vi "Initialize Hardware.vi"(8 "error in (no error)":errorcluster, 9 "Connection Setting":T1={"Connection Ref"=variant, "Serial Configuration"={"Baud Rate"=9600}} {"Serial Configuration"."Baud Rate" items=["300"=300, "600"=600, "1200"=1200, "2400"=2400, "4800"=4800, "9600"=9600, "19200"=19200]}, 10 "DAQ Type":enum16{"Hardware", "Simulation"}(ring), 11 "BK-Precision in":refnum<class "BK-Precision.lvclass">) -> (0 "error out":errorcluster, 3 "BK-Precision out":refnum<class "BK-Precision.lvclass">)   [LabVIEW 2021, in "DC PWS.lvlib" / "BK-Precision.lvclass"]
uses:
  BK-Precision.lvclass
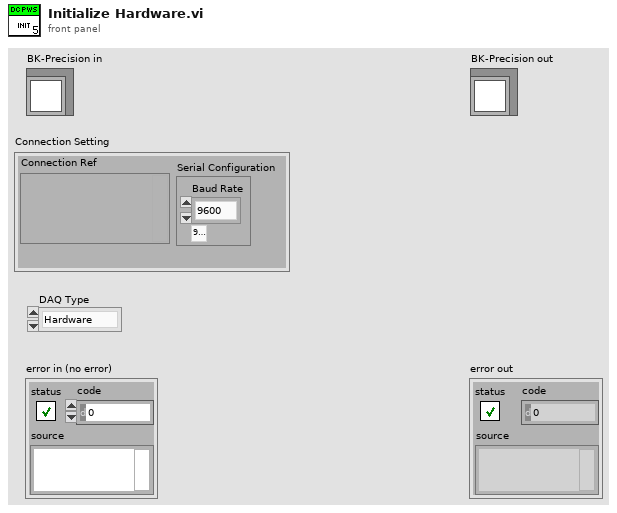
[diagram p1: front panel]
types:
  T1 = cluster{"Connection Ref":variant, "Serial Configuration":cluster{"Baud Rate":u32}}
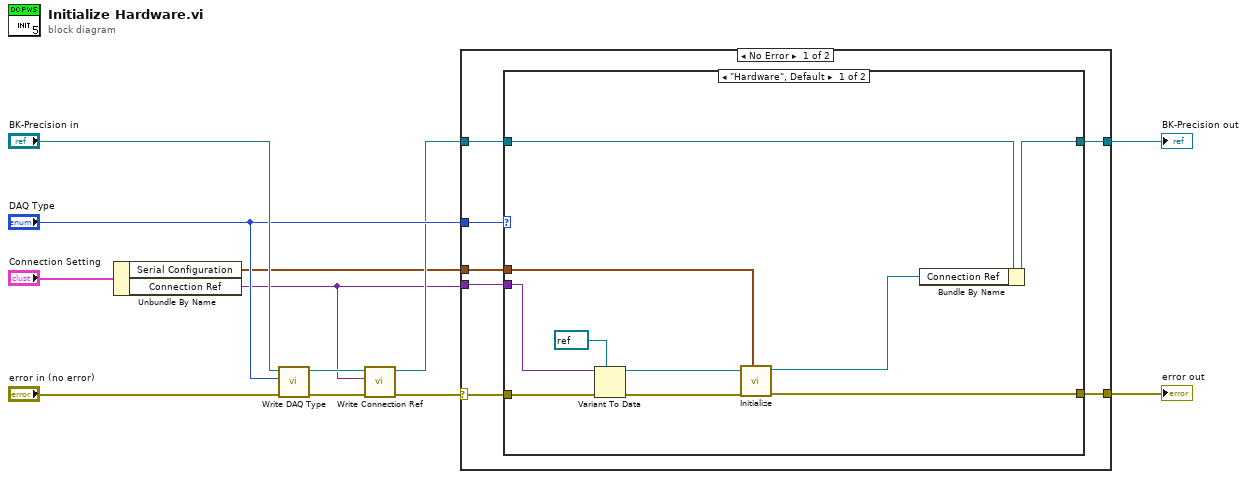
[diagram p0: block diagram]
diagram:
  n1 = Unbundle By Name("Connection Setting") -> ("Serial Configuration"=w1:cluster{"Baud Rate":u32}, "Connection Ref"=w2:variant)
  n2 = call "Write DAQ Type.vi"("error in (no error)"="error in (no error)", "Type"="DAQ Type", "BK-Precision in"="BK-Precision in") -> ("error out"=w9:errorcluster, "BK-Precision out"=w8:refnum<class "BK-Precision.lvclass">)  [unwired: 7 in]
  n3 = call "Write Connection Ref.vi"("error in (no error)"=w9, "Conn Ref"=w2, "BK-Precision in"=w8) -> ("error out"=w6:errorcluster, "BK-Precision out"=w7:refnum<class "BK-Precision.lvclass">)  [unwired: 7 in]
  n4 = case shown="No Error" w6 {
    selector: w6 -> [w16 w33]
    tunnel: "DAQ Type" -> [w19 _]
    tunnel: w7 -> [w18 w32]
    tunnel: w2 -> [w17 _]
    tunnel: [w15 w33] -> w5
    tunnel: [w14 w32] -> w4
    tunnel: w1 -> [w13 _]
    frame No Error {
      n5 = case shown="\"Hardware\", Default" w19 {
        tunnel: w18 -> [w23 w31]
        tunnel: w17 -> [w27 _]
        tunnel: w16 -> [w29 w30]
        tunnel: [w24 w30] -> w15
        tunnel: [w22 w31] -> w14
        tunnel: w13 -> [w20 _]
        frame "Hardware", Default {
          n6 = Variant To Data(error in=w29, type=refnum<visa-resource-name> refnum ("VISA resource name"), Variant=w27) -> (data=w25:refnum<visa-resource-name>, error out=w26:errorcluster)
          n7 = call <instrlib>:"Initialize.vi"("Serial Configuration"=w20, "error in (no error)"=w26, "VISA resource name"=w25) -> ("error out"=w24:errorcluster, "VISA resource name out"=w21:refnum<visa-resource-name>)  [unwired: 7 in]
          n8 = Bundle By Name(cluster=w23, "Connection Ref"=w21) -> (w22:refnum<class "BK-Precision.lvclass">)
        }
        frame "Simulation" {
        }
      }
    }
    frame Error {
    }
  }
  "error out" <- w5
  "BK-Precision out" <- w4
